vi "Get CD Item Property Value.vi"(8 "error in (no error)":errorcluster, 10 "CD Item Ref in":T1 format="%.0x", 11 "I32 Parameter in":refnum<class "I32 Parameter.lvclass">) -> (0 "error out":errorcluster, 3 "I32 Parameter out":refnum<class "I32 Parameter.lvclass">)   [LabVIEW 2019, in "CD Parameter Manager API.lvlib" / "I32 Parameter.lvclass"]
uses:
  I32 Parameter.lvclass
  C:/Repositories/UI-Control-Initializer-API/Source/Parameter Class/Parameter.lvclass
  <vilib>/NI VeriStand/Custom Device API/Custom Device Item Ref.ctl
  Parameter Class/Parameter.lvclass/Parameter.ctl
  I32 Parameter.lvclass/I32 Parameter.ctl
  Parameter Class/Member Accessors/Read Control label.vi
  Member Accessors/Read Value.vi
  Member Accessors/Write Value.vi
  <vilib>/NI VeriStand/Custom Device API/Get Item Property (I32).vi
  <vilib>/NI VeriStand/Custom Device API/Custom Device API.lvlib
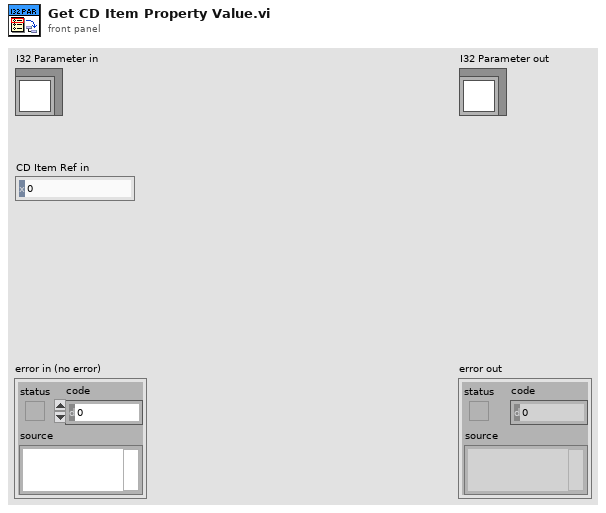
[diagram p1: front panel]
types:
  T1 = typedef "Custom Device API.lvlib/Custom Device Item Ref.ctl" = u64
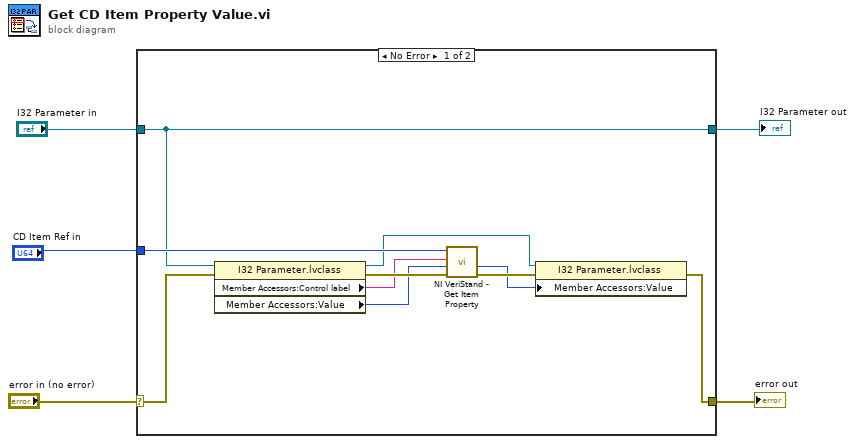
[diagram p0: block diagram]
diagram:
  n1 = case shown="No Error" "error in (no error)" {
    selector: "error in (no error)" -> [w14 w16]
    tunnel: [w9 w16] -> w4
    tunnel: "CD Item Ref in" -> [w15 _]
    tunnel: [w7 w17] -> w2
    tunnel: "I32 Parameter in" -> [w7 w17]
    frame No Error {
      n2 = property class="I32 Parameter.lvclass"(reference=w7, error in=w14) -> (reference out=w6:refnum<class "I32 Parameter.lvclass">, error out=w13:errorcluster, "Member Accessors:Control label"=w12:string, "Member Accessors:Value"=w11:i32)
      n3 = call-poly <vilib>:"NI VeriStand - Get Item Property.vi"("error in (no error)"=w13, "Default Value"=w11, "Property Name"=w12, "Item Ref in"=w15) -> ("error out"=w10:errorcluster, "Value"=w8:i32)  [unwired: 4 in, 2 out]
      n4 = property class="I32 Parameter.lvclass"(reference=w6, error in=w10, "Member Accessors:Value"=w8) -> (error out=w9:errorcluster)  [unwired: 1 out]
    }
    frame Error {
    }
  }
  "error out" <- w4
  "I32 Parameter out" <- w2
